vi "TEMPLATE After.vi"(6 "Teller":T3 {"Absolute Time" format="%<%x %.3X>T"}, 8 "Error in":errorcluster, 9 "Metadata in":T2, 10 "Data in":T1, 11 "TEMPLATE jettl Msg in":refnum<class "TEMPLATE jettl Msg.lvclass">) -> (0 "Error out":errorcluster, 1 "Metadata out":T2, 2 "Data out":T1, 3 "TEMPLATE jettl Msg out":refnum<class "TEMPLATE jettl Msg.lvclass">)   [LabVIEW 2020, in "_Template.lvlib" / "Templates.lvlib" / "TEMPLATE jettl Msg.lvlib" / "TEMPLATE jettl Msg.lvclass"]
uses:
  TEMPLATE jettl Msg.lvclass
  jettl/jettl/Unified Actor Relation.ctl
  jettl/jettl/jettl.lvlib
  jettl/jettl/Teller.ctl
  Metadata.ctl
  TEMPLATE jettl Msg.lvlib
  Data.ctl
panel:
  # "This front panel should not be manipulated."
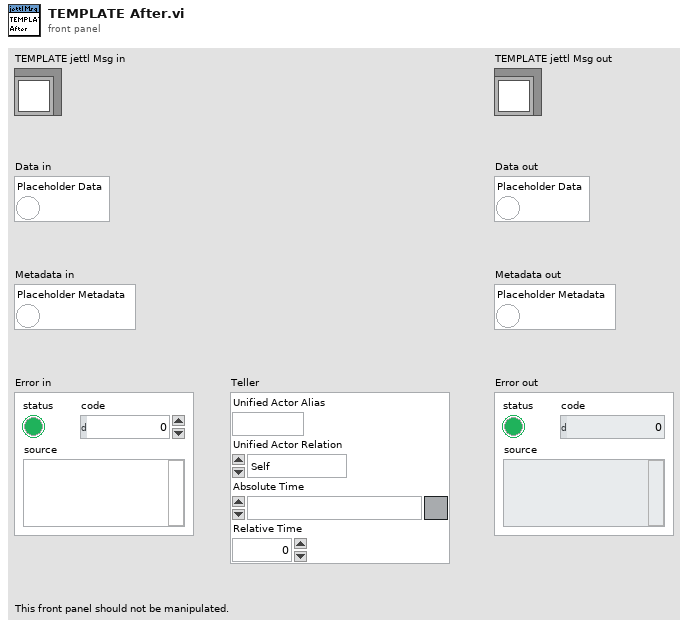
[diagram p1: front panel]
types:
  T1 = typedef "_Template.lvlib/Templates.lvlib/TEMPLATE jettl Msg.lvlib/Data.ctl" = cluster{"Placeholder Data":bool}
  T2 = typedef "_Template.lvlib/Templates.lvlib/TEMPLATE jettl Msg.lvlib/Metadata.ctl" = cluster{"Placeholder Metadata":bool}
  T3 = typedef "jettl.lvlib/Teller.ctl" = cluster{"Unified Actor Alias":string, "Unified Actor Relation":T4, "Absolute Time":timestamp, "Relative Time":dbl}
  T4 = typedef "jettl.lvlib/Unified Actor Relation.ctl" = enum16{"Self", "Parent", "Child"}
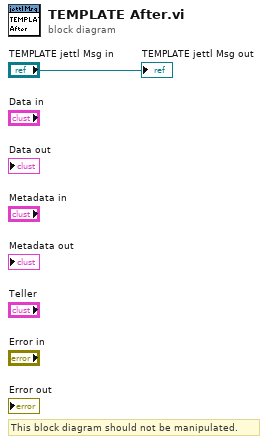
[diagram p0: block diagram]
diagram:
  # "This block diagram should not be manipulated."
  "TEMPLATE jettl Msg out" <- "TEMPLATE jettl Msg in"
